vi "Inspect.vi"(7 "Actor in":refnum<class "Actor.lvclass">, 8 "Error in":errorcluster, 9 "Msg":refnum<class "Msg.lvclass">, 10 "Within Unified Msgs":bool) -> (2 "Proceed":bool=TRUE, 5 "Actor out":refnum<class "Actor.lvclass">)   [LabVIEW 2025, in "jettl.lvlib"]
uses:
  jettl.lvlib
  Msg/Msg.lvclass
  Actor/Actor.lvclass
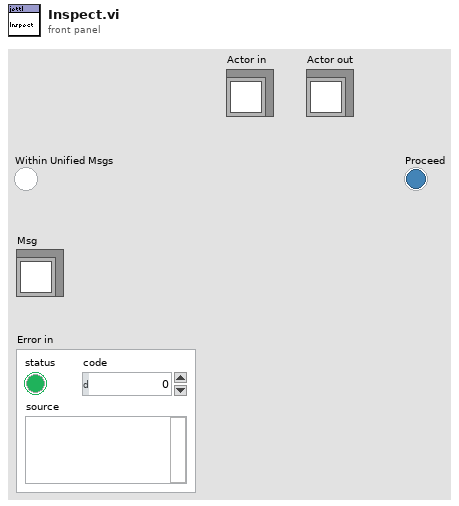
[diagram p1: front panel]
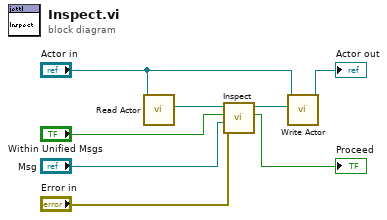
[diagram p0: block diagram]
diagram:
  n1 = call-dynamic "Read Actor.vi"("Actor in"="Actor in") -> ("Actor"=w8:refnum<class "Actor.lvclass">)  [unwired: 10 in]
  n2 = call-dynamic "Inspect.vi"("Error in"="Error in", "Msg"="Msg", "Within Unified Msgs"="Within Unified Msgs", "Actor in"=w8) -> ("Proceed"=→"Proceed":bool, "Actor out"=w7:refnum<class "Actor.lvclass">)  [unwired: 6 in]
  n3 = call-dynamic "Write Actor.vi"("Actor"=w7, "Actor in"="Actor in") -> ("Actor out"=→"Actor out":refnum<class "Actor.lvclass">)  [unwired: 9 in]
